vi "Set Embedded Data Logger FIFO Depth.vi"(8 "error in":errorcluster, 10 "fifo depth":i32, 11 "embedded data logger in":T1 format="%.0x") -> (0 "error out":errorcluster, 3 "embedded data logger out":T1 format="%.0x")   [LabVIEW 2027, in "Embedded Data Logger Scripting.lvlib"]
uses:
  Embedded Data Logger Scripting.lvlib
  <vilib>/NI VeriStand/Custom Device API/Custom Device Item Ref.ctl
  <vilib>/NI VeriStand/Custom Device API/Set Item Property (I32).vi
  <vilib>/NI VeriStand/Custom Device API/Custom Device API.lvlib
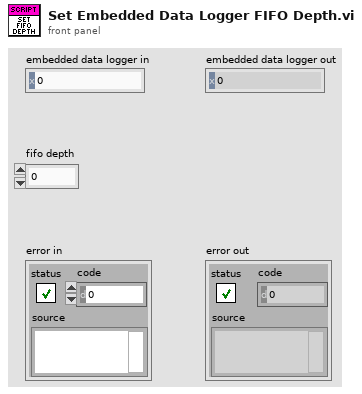
[diagram p1: front panel]
types:
  T1 = typedef "Custom Device API.lvlib/Custom Device Item Ref.ctl" = u64
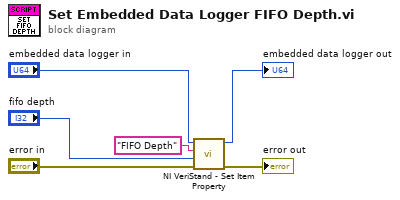
[diagram p0: block diagram]
diagram:
  n1 = call-poly <vilib>:"NI VeriStand - Set Item Property.vi"("error in (no error)"="error in", "Value"="fifo depth", "Property Name"="FIFO Depth", "Item Ref in"="embedded data logger in") -> ("error out"=→"error out":errorcluster, "Item Ref out"=→"embedded data logger out":T1)  [unwired: 6 out]
